vi "DynamicRegistration1.vi"() -> ()   [LabVIEW 2020]
panel:
  in  "Ring":u16(ring)
  in  "stop":bool
  out "Iiterations":i32
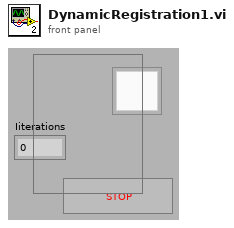
[diagram p1: front panel]
types:
  T1 = typedef "LVPoint32TypeDef.ctl" = cluster{"Horizontal":i32, "Vertical":i32}
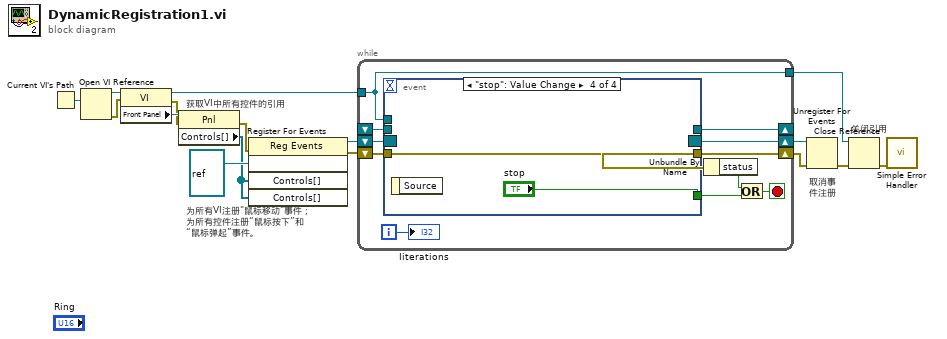
[diagram p0: block diagram]
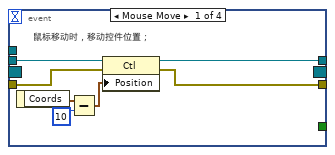
[diagram p2: hidden frame]
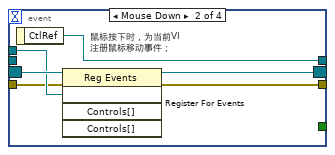
[diagram p3: hidden frame]
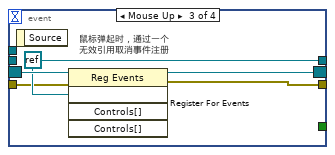
[diagram p4: hidden frame]
diagram:
  # "关闭引用"
  # "取消事\n件注册"
  # "为所有VI注册\"鼠标移动\"事件；\n为所有控件注册“鼠标按下”和\n“鼠标弹起”事件。"
  # "获取VI中所有控件的引用"
  n1 = Current VI's Path() -> (path=w14:path)
  n2 = Open VI Reference(vi path=w14) -> (vi reference=w1:refnum<vi>, error out=w13:errorcluster)  [unwired: 1 in, 4 out]
  n3 = property class="VI"(reference=w1, error in=w13) -> (error out=w11:errorcluster, "Front Panel"=w12:refnum<vi>)  [unwired: 1 out]
  n4 = property class="Pnl"(reference=w12, error in=w11) -> (error out=w6:errorcluster, "Controls[]"=w7:refnum<vi>[])  [unwired: 1 out]
  n5 = register-events(error in=w6, refnum<vi> refnum, w7, w7) -> (reference out=w15:refnum<event-registration>, error out=w5:errorcluster)  [unwired: 1 in]
  n6 = while {
    shift-right: [w24] -> _
    shift-left: _ -> [w23]
    tunnel: [w16] -> w9
    shift-right: [w22] -> w10
    shift-left: w15 -> [w25]
    shift-right: [w17] -> w4
    shift-left: w5 -> [w21]
    tunnel: w1 -> [w16]
    i -> [w26]
    stop <- w19 stop-if-true
    n7 = event shown="[3] \"stop\": Value Change" {
      selector: w25 -> [_ w39 w44 _]
      dyn-events: [_ w37 w42 _] -> w22
      timeout: _ -> [_ _ _ _]
      tunnel: [_ _ _ "stop"] -> w18
      tunnel: w16 -> [_ w38 _ _]
      tunnel: [w29 w34 w43 _] -> w24
      tunnel: w23 -> [w30 _ _ _]
      tunnel: w21 -> [w28 w36 w41 w45]
      tunnel: [w27 w35 w40 w45] -> w17
      event Mouse Move {
        # "鼠标移动时，移动控件位置；"
        n8 = event-data() -> ("Coords"=w33:T1)  [unwired: 1 out]
        n9 = Subtract(x=w33, y=10) -> (x-y=w31:T1)
        n10 = property on="Property Node" class="Ctl"(reference=w30, error in=w28, "Position"=w31) -> (reference out=w29:refnum<vi>, error out=w27:errorcluster)
      }
      event Mouse Down {
        # "鼠标按下时，为当前VI\n注册鼠标移动事件；"
        n11 = event-data() -> ("CtlRef"=w34:refnum<vi>)  [unwired: 1 out]
        n12 = register-events(reference=w39, error in=w36, w38) -> (reference out=w37:refnum<event-registration>, error out=w35:errorcluster)  [unwired: 2 out]
      }
      event Mouse Up {
        w43 = refnum<k0> refnum
        # "鼠标弹起时，通过一个\n无效引用取消事件注册"
        n13 = event-data() -> ()  [unwired: 2 out]
        n14 = register-events(reference=w44, error in=w41, w43) -> (reference out=w42:refnum<event-registration>, error out=w40:errorcluster)  [unwired: 2 out]
      }
      event "stop": Value Change {
        n15 = event-data() -> ()  [unwired: 2 out]
      }
    }
    n16 = Unbundle By Name(w17) -> ("status"=w20:bool)
    n17 = Or(x=w20, y=w18) -> (x .or. y?=w19:bool)
    "Iiterations" <- w26
  }
  n18 = Unregister For Events(event registration refnum=w10, error in=w4) -> (error out=w3:errorcluster)
  n19 = Close Reference(reference=w9, error in (no error)=w3) -> (error out=w2:errorcluster)
  n20 = call <vilib>:"Simple Error Handler.vi"("error in (no error)"=w2) -> ()  [unwired: 1 in, 8 out]
